vi "按钮移动.vi"() -> ()   [LabVIEW 2018]
panel:
  in  "停止":bool
  in  "左":bool
  in  "右":bool
  in  "上":bool
  in  "下":bool
  out "布尔":bool
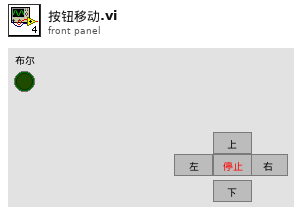
[diagram p1: front panel]
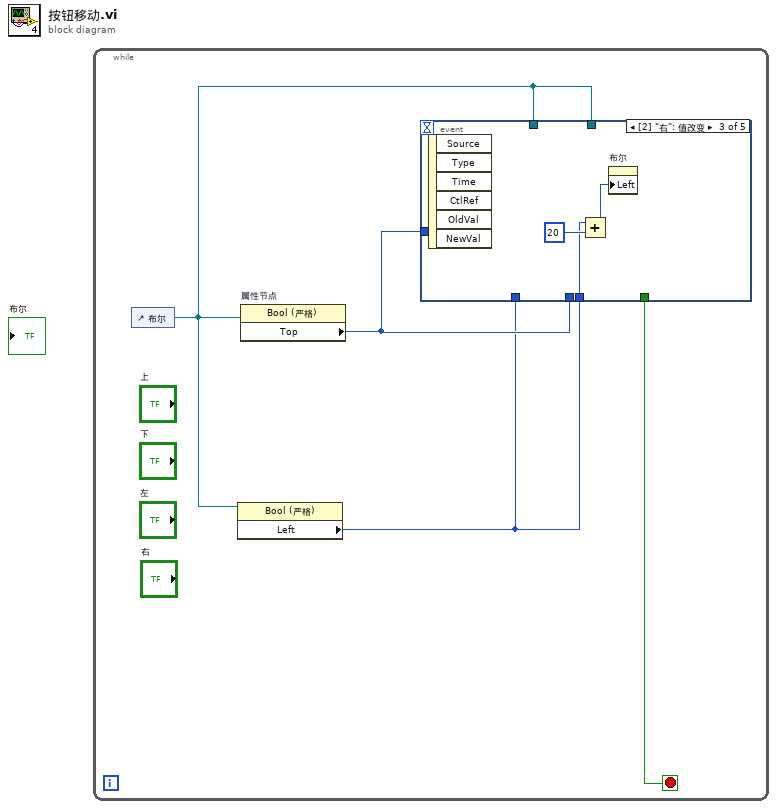
[diagram p0: block diagram]
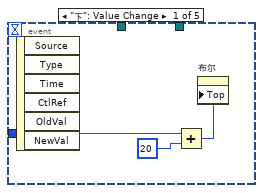
[diagram p2: hidden frame]
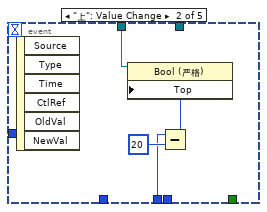
[diagram p3: hidden frame]
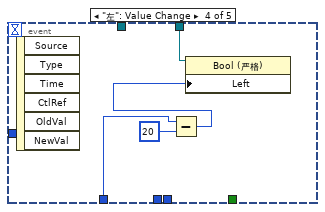
[diagram p4: hidden frame]
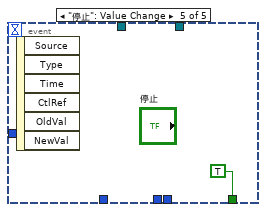
[diagram p5: hidden frame]
diagram:
  n1 = while {
    stop <- w2 stop-if-true
    n2 = control-ref of="布尔"() -> (w1:refnum<vi>)
    n3 = property class="Bool (严格)"(reference=w1) -> ("Left"=w3:i32)  [unwired: 1 in, 2 out]
    n4 = property on="属性节点" class="Bool (严格)"(reference=w1) -> ("Top"=w4:i32)  [unwired: 1 in, 2 out]
    n5 = event shown="[2] \"右\": 值改变" {
      selector: _ -> [_ _ _ _ _]
      dyn-events: _ -> [_ _ _ _ _]
      timeout: _ -> [_ _ _ _ _]
      tunnel: w4 -> [w6 _ _ _ _]
      tunnel: w4 -> [_ w10 _ _ _]
      tunnel: w3 -> [_ _ w13 _ _]
      tunnel: w3 -> [_ _ _ w17 _]
      tunnel: [_ _ _ _ TRUE] -> w2
      tunnel: w1 -> [_ w8 _ _ _]
      tunnel: w1 -> [_ _ _ w15 _]
      event "下": Value Change {
        n6 = event-data() -> ()  [unwired: 1 in, 6 out]
        n7 = Add(x=w6, y=20) -> (x+y=w5:i32)
        n8 = property on="布尔" class="Bool (严格)"("Top"=w5) -> ()  [unwired: 2 in, 2 out]
      }
      event "上": Value Change {
        n9 = event-data() -> ()  [unwired: 1 in, 6 out]
        n10 = Subtract(x=w10, y=20) -> (x-y=w9:i32)
        n11 = property on="属性节点" class="Bool (严格)"(reference=w8, "Top"=w9) -> ()  [unwired: 1 in, 2 out]
      }
      event "右": Value Change {
        n12 = event-data() -> ()  [unwired: 1 in, 6 out]
        n13 = Add(x=w13, y=20) -> (x+y=w12:i32)
        n14 = property on="布尔" class="Bool (严格)"("Left"=w12) -> ()  [unwired: 2 in, 2 out]
      }
      event "左": Value Change {
        n15 = event-data() -> ()  [unwired: 1 in, 6 out]
        n16 = Subtract(x=w17, y=20) -> (x-y=w16:i32)
        n17 = property on="属性节点" class="Bool (严格)"(reference=w15, "Left"=w16) -> ()  [unwired: 1 in, 2 out]
      }
      event "停止": Value Change {
        n18 = event-data() -> ()  [unwired: 1 in, 6 out]
      }
    }
  }
